vi "TurtleModeSailSuggestion.vi"(4 "OLD Suggested Rudder Setpoint":T2 min=-1.0 max=1.0, 6 "OLD Suggested Sail Setpoints":T3 {"MainSailSuggestion" min=0.0 max=1.0; "JibSailSuggestion" min=0.0 max=1.0}, 9 "AbsoluteWindAngle":dbl, 10 "BoatVectorVelocity":T1, 11 "RelativeWindAngle":dbl) -> (2 "Suggested Rudder Setpoint":T2 min=-1.0 max=1.0, 3 "Suggested Sail Setpoints":T3 {"MainSailSuggestion" min=0.0 max=1.0; "JibSailSuggestion" min=0.0 max=1.0})   [LabVIEW 2013]
doc: "Suggests sail and rudder settings that will keep the boat safe in high winds.\n\nThis should most likely be done by trying to keep the sails perpendicular to the wind and maybe using the rudder to turn the boat into the wind when possible. Locking the rudder in place is also a possibility.\n\nEric Schneider and Bonnie Ishiguro, Jan. 2014"
uses:
  Data/TypeDefs/Rudder Set Suggestions.ctl
  Data/TypeDefs/Sail Set Suggestions.ctl
panel:
  # "Suggests sail and rudder settings that\nwill keep the boat safe in high winds.\n\nTODO: his should most likely be done by trying\nto keep the sails perpendicular to the wind\nand maybe using the rudder to turn the\nboat into the wind when possible. Locking\nthe rudder in place is also a possibility.\n\nThe decision for whether to go into turtle mode\nis NOT made here, that is done in\nDetermineStateOfBoat.vi"
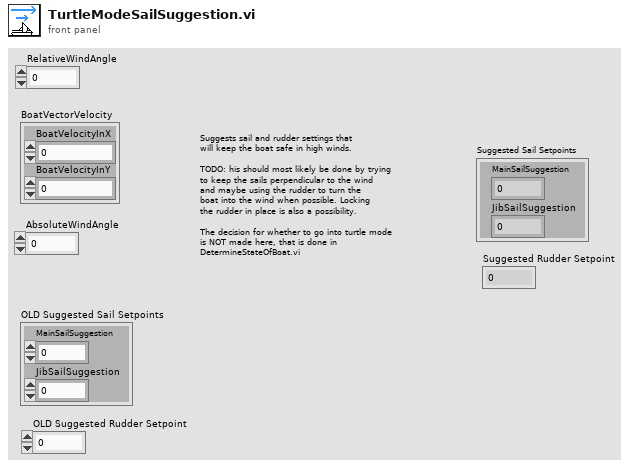
[diagram p1: front panel]
types:
  T1 = cluster{"BoatVelocityInY":dbl, "BoatVelocityInX":dbl}
  T2 = typedef "Rudder Set Suggestions.ctl" = dbl
  T3 = typedef "Sail Set Suggestions.ctl" = cluster{"MainSailSuggestion":dbl, "JibSailSuggestion":dbl}
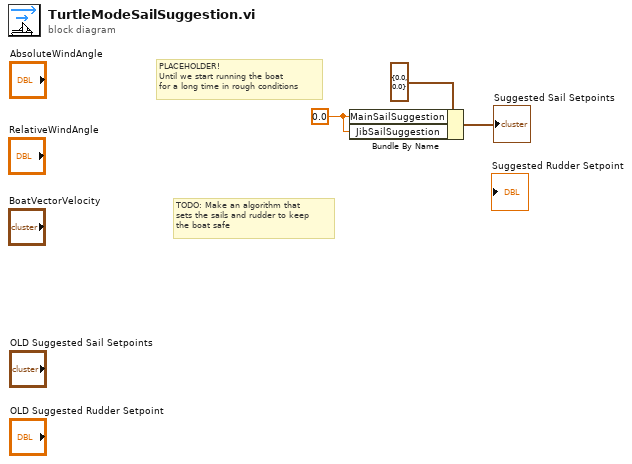
[diagram p0: block diagram]
diagram:
  w1 = 0.0 ("MainSailSuggestion")
  # "PLACEHOLDER!\nUntil we start running the boat\nfor a long time in rough conditions"
  # "TODO: Make an algorithm that\nsets the sails and rudder to keep\nthe boat safe"
  n1 = Bundle By Name(cluster=T3 {"MainSailSuggestion"=0.0, "JibSailSuggestion"=0.0} ("output cluster"), "MainSailSuggestion"=w1, "JibSailSuggestion"=w1) -> (→"Suggested Sail Setpoints":T3)
